vi "comm termination2.vi"(8 "error in (no error)":errorcluster, 9 "termination":string, 10 "Termination Mode":enum16{"none", "chars", "string", "regex"}(ring), 11 "Comm Handle":u32) -> (0 "error out":errorcluster, 3 "dup Comm Handle":u32)   [LabVIEW 2017, in "lvserial.lvlib"]
doc: "Configures the termiation characters for the serial port."
uses:
  lvserial.lvlib
  lvserial.dll
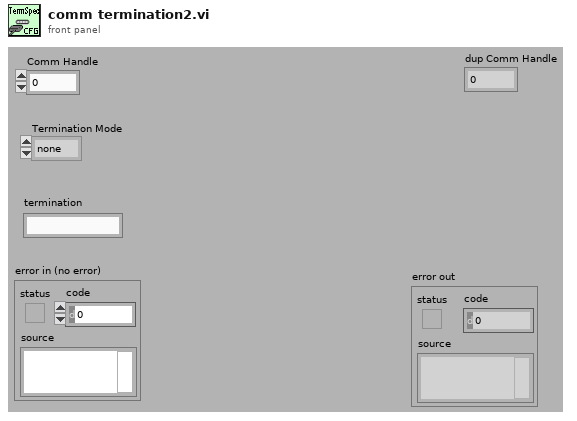
[diagram p1: front panel]
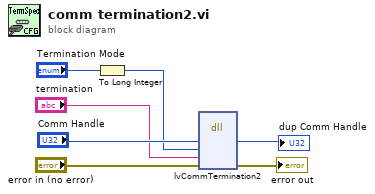
[diagram p0: block diagram]
diagram:
  n1 = To Long Integer(number="Termination Mode") -> (32bit integer=w1:i32)
  n2 = dll-call lib="lvserial.dll" fn="lvCommTermination2"("hComm"="Comm Handle", "lTerminationMode"=w1, "shTermination"="termination", "error in (no error)"="error in (no error)") -> ("hComm"=→"dup Comm Handle":u32, "error in (no error)"=→"error out":errorcluster)  [unwired: 5 in, 3 out]
